vi "StockFPGA_InlinedAdjustHostInterfaceError.vi"(11 "error in":errorcluster, 12 "prior error in":errorcluster, 13 "node name for error reporting":T2, 14 "what happens to top level VI":T1) -> (15 "error out":errorcluster)   [LabVIEW 2019]
uses:
  <vilib>/rvi/interface/common/niFpgaNodeNameForErrorReporting.ctl
  <vilib>/rvi/errors/niLvFpgaWhatHappensToTopLevelVI.ctl
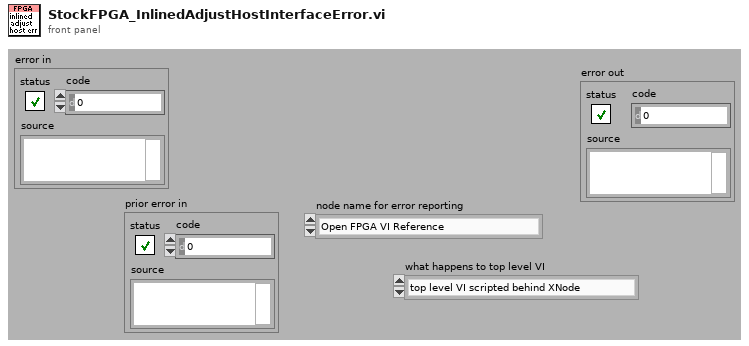
[diagram p1: front panel]
types:
  T1 = typedef "niLvFpgaWhatHappensToTopLevelVI.ctl" = enum16{"top level VI scripted behind XNode", "top level VI inlined behind XNode"}
  T2 = typedef "niFpgaNodeNameForErrorReporting.ctl" = enum16{"Open FPGA VI Reference", "Read/Write Control", "Invoke Method: Abort", "Invoke Method: Acknowledge IRQ", "Invoke Method: Download", "Invoke Method: FIFO.Configure", "Invoke Method: FIFO.Read", "Invoke Method: FIFO.Start", "Invoke Method: FIFO.Stop", "Invoke Method: FIFO.Write", "Invoke Method: Reset", "Invoke Method: Run", "Invoke Method: Wait on IRQ", "Close FPGA VI Reference", "Invoke Method: FIFO.Acquire Read Region", "Invoke Method: FIFO.Acquire Write Region"}
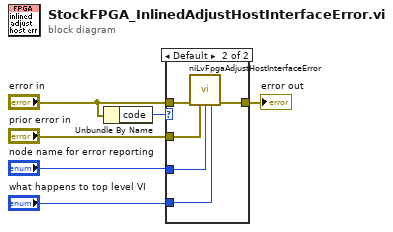
[diagram p0: block diagram]
diagram:
  n1 = Unbundle By Name("error in") -> ("code"=w2:i32)
  n2 = case shown="Default" w2 {
    tunnel: [w7 w12] -> w3
    tunnel: "prior error in" -> [w7 w11]
    tunnel: "what happens to top level VI" -> [_ w10]
    tunnel: "node name for error reporting" -> [_ w9]
    tunnel: "error in" -> [_ w8]
    frame 0 {
    }
    frame Default {
      n3 = call <vilib>:"niLvFpgaAdjustHostInterfaceError.vi"("error in"=w8, "prior error in"=w11, "node name for error reporting"=w9, "what happens to top level VI"=w10) -> ("error out"=w12:errorcluster)  [unwired: 11 in]
    }
  }
  "error out" <- w3
